vi "someraph.vi"() -> ()   [LabVIEW 2019]
uses:
  <vilib>/Utility/file.llb/Read Delimited Spreadsheet (DBL).vi
panel:
  out "XY Graph":cluster{"all rows":dbl[], "all rows":dbl[]}(graph)
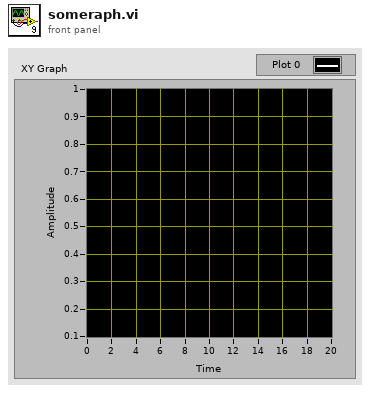
[diagram p1: front panel]
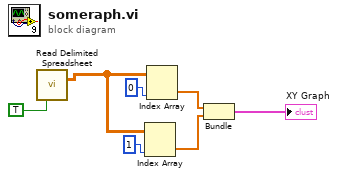
[diagram p0: block diagram]
diagram:
  n1 = call-poly <vilib>:"Read Delimited Spreadsheet.vi"("transpose? (F)"=TRUE) -> ("all rows"=w7:dbl[][])  [unwired: 9 in, 5 out]
  n2 = Index Array(array=w7, index (col)=1 ("index (row)")) -> (element=w5:dbl[])  [unwired: 1 in]
  n3 = Index Array(array=w7, index (col)=0 ("index (row)")) -> (element=w6:dbl[])  [unwired: 1 in]
  n4 = Bundle("all rows"=w6, "all rows"=w5) -> (→"XY Graph":cluster{"all rows":dbl[], "all rows":dbl[]})  [unwired: 1 in]
